vi "Emballage_BDD_Lecture_table_EMB_FAMILLE_VALVE.vi"(8 "entrée d'erreur (pas d'erreur)":errorcluster) -> (0 "sortie d'erreur":errorcluster, 3 "données":string[][](array[string]))   [LabVIEW 2020]
uses:
  Modules/FS/60_FS_Controles/60_FS_SetGet.ctl
  <vilib>/addons/database/Connection.llb/DB Tools Open Connec (Path).vi
  <vilib>/addons/database/Connection.llb/Conn Execute.vi
  <vilib>/addons/database/Recordset.llb/Rec Fetch Recordset Data (R).vi
  <vilib>/addons/database/Recordset.llb/Rec Destroy - Connection.vi
  <vilib>/addons/database/NI_Database_API.lvlib
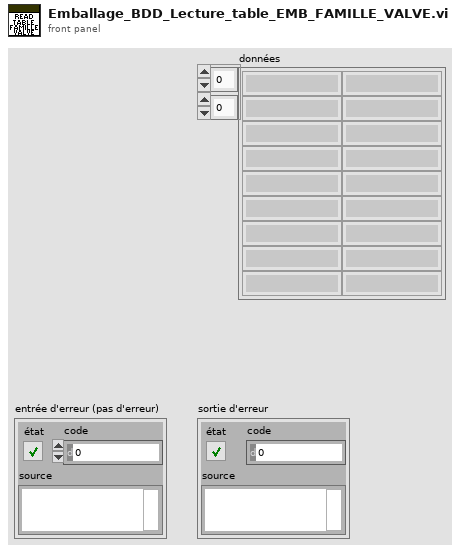
[diagram p1: front panel]
types:
  T1 = typedef "60_FS_SetGet.ctl" = enum16{"set", "get"}
  T2 = typedef "60_FS_CLT_Chemins.ctl" = cluster{"Racine_local":path, "Racine_reseau":path, "Racine_Support_Application":path, "Fichier_Journalisation":path, "Connexion_BDD_VSX":path, "Connexion_BDD_PLZ":path}
  T3 = typedef "NI_Database_API.lvlib/Conn ObjectReference.ctl" = refnum<k1>
  T4 = typedef "NI_Database_API.lvlib/Rec ObjectReference.ctl" = refnum<k1>
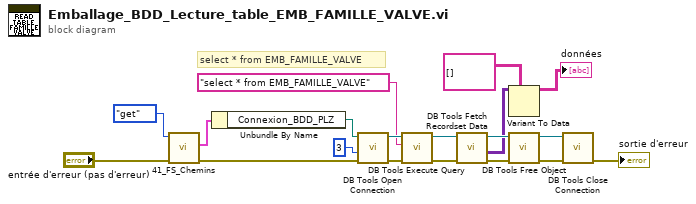
[diagram p0: block diagram]
diagram:
  # "select * from EMB_FAMILLE_VALVE"
  n1 = call "41_FS_Chemins.vi"("error in (no error)"="entrée d'erreur (pas d'erreur)", "SetGet"=60_FS_SetGet."get") -> ("error out"=w4:errorcluster, "CLT_Chemins_out"=w2:T2)  [unwired: 8 in]
  n2 = Unbundle By Name(w2) -> ("Connexion_BDD_PLZ"=w1:path)
  n3 = call-poly <vilib>:"DB Tools Open Connection.vi"("error in (no error)"=w4, "connection timeout (15)"=3, "connection information"=w1) -> ("error out"=w14:errorcluster, "connection reference"=w13:T3)  [unwired: 5 in]
  n4 = call-poly <vilib>:"DB Tools Execute Query.vi"("error in (no error)"=w14, "SQL query"="select * from EMB_FAMILLE_VALVE", "connection reference"=w13) -> ("error out"=w8:errorcluster, "recordset reference"=w11:T4)  [unwired: 5 in]
  n5 = call-poly <vilib>:"DB Tools Fetch Recordset Data.vi"("error in (no error)"=w8, "recordset reference"=w11) -> ("error out"=w16:errorcluster, "recordset data"=w9:variant[][], "recordset reference out"=w18:T4)  [unwired: 3 in]
  n6 = Variant To Data(type=string[][] [] ("Liste des champs à lire 2"), Variant=w9) -> (data=→"données":string[][])  [unwired: 1 in, 1 out]
  n7 = call-poly <vilib>:"DB Tools Free Object.vi"("error in (no error)"=w16, "recordset reference"=w18) -> ("error out"=w17:errorcluster, "connection reference"=w19:T3)  [unwired: 8 in]
  n8 = call <vilib>:"DB Tools Close Connection.vi"("error in (no error)"=w17, "connection reference"=w19) -> ("error out"=→"sortie d'erreur":errorcluster)  [unwired: 5 in]
